vi "zadanie_1.vi"() -> ()   [LabVIEW 2017]
panel:
  out "0 Hz 2":bool
  out "2 Hz 2":bool
  out "1 Hz 2":bool
  in  "stop":bool
  out "wybr_czest":enum16{"0 Hz", "1 Hz", "2 Hz"}(ring)
  in  "2 Hz":bool
  in  "1 Hz":bool
  in  "0 Hz":bool
  out "dioda":bool
  # "Wybrana czestotliwosc"
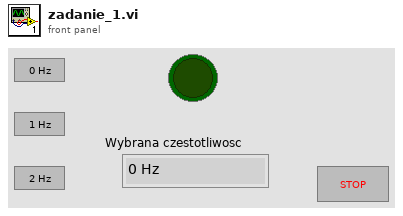
[diagram p1: front panel]
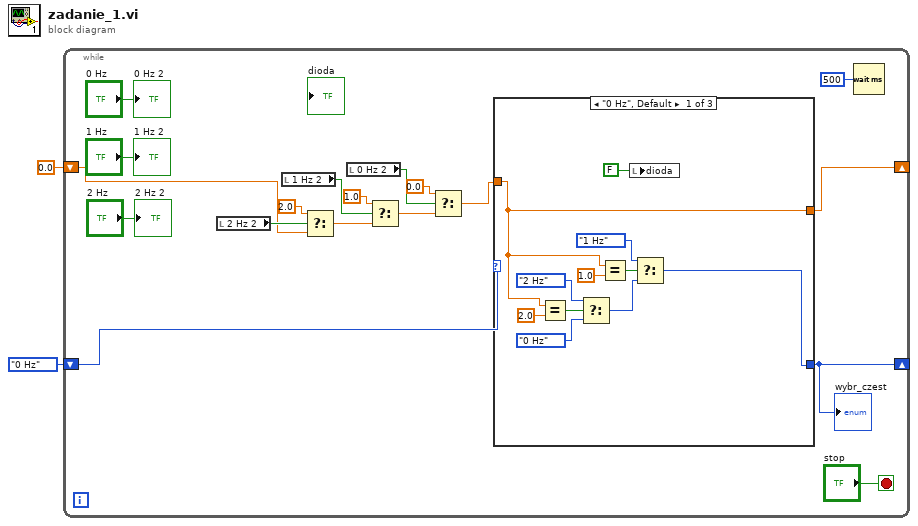
[diagram p0: block diagram]
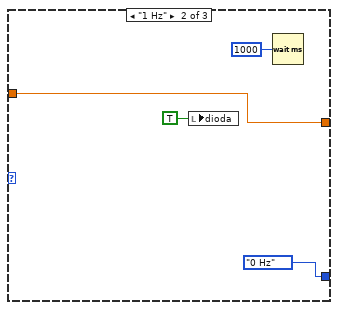
[diagram p2: hidden frame]
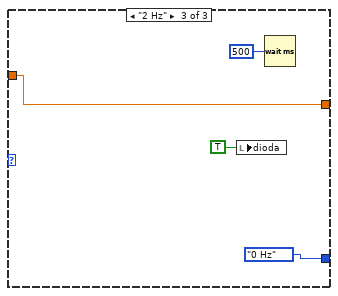
[diagram p3: hidden frame]
diagram:
  n1 = while {
    shift-right: [w3] -> _
    shift-left: enum16{"0 Hz", "1 Hz", "2 Hz"}."0 Hz" -> [w18]
    shift-right: [w17] -> _
    shift-left: 0.0 ("Numeric") -> [w11]
    stop <- "stop" stop-if-true
    n2 = local read "2 Hz 2"() -> (w16:bool)
    n3 = local read "1 Hz 2"() -> (w14:bool)
    n4 = Select(t=2.0, s=w16, f=w11) -> (s? t:f=w15:dbl)
    n5 = local read "0 Hz 2"() -> (w8:bool)
    n6 = Select(t=1.0, s=w14, f=w15) -> (s? t:f=w10:dbl)
    n7 = Select(t=0.0, s=w8, f=w10) -> (s? t:f=w7:dbl)
    n8 = case shown="\"0 Hz\", Default" w18 {
      tunnel: [w30 enum16{"0 Hz", "1 Hz", "2 Hz"}."0 Hz" enum16{"0 Hz", "1 Hz", "2 Hz"}."0 Hz"] -> w3
      tunnel: [w24 w33 w37] -> w17
      tunnel: w7 -> [w24 w33 w37]
      frame "0 Hz", Default {
        n9 = Equal?(x=w24, y=2.0) -> (x = y?=w25:bool)
        n10 = Select(t=enum16{"0 Hz", "1 Hz", "2 Hz"}."2 Hz", s=w25, f=enum16{"0 Hz", "1 Hz", "2 Hz"}."0 Hz") -> (s? t:f=w29:enum16{"0 Hz", "1 Hz", "2 Hz"})
        n11 = Equal?(x=w24, y=1.0) -> (x = y?=w27:bool)
        n12 = local write "dioda"(FALSE ("Boolean")) -> ()
        n13 = Select(t=enum16{"0 Hz", "1 Hz", "2 Hz"}."1 Hz", s=w27, f=w29) -> (s? t:f=w30:enum16{"0 Hz", "1 Hz", "2 Hz"})
      }
      frame "1 Hz" {
        n14 = local write "dioda"(TRUE ("Boolean")) -> ()
        n15 = Wait (ms)(milliseconds to wait=u32 1000) -> ()  [unwired: 1 out]
      }
      frame "2 Hz" {
        n16 = local write "dioda"(TRUE ("Boolean")) -> ()
        n17 = Wait (ms)(milliseconds to wait=u32 500) -> ()  [unwired: 1 out]
      }
    }
    "wybr_czest" <- w3
    n18 = Wait (ms)(milliseconds to wait=u32 500) -> ()  [unwired: 1 out]
    "1 Hz 2" <- "1 Hz"
    "2 Hz 2" <- "2 Hz"
    "0 Hz 2" <- "0 Hz"
  }
